vi "SyntaxClean.vi"(8 "error in (no error)":errorcluster, 11 "Logical Parsed Expression":T1) -> (0 "error out":errorcluster, 3 "Logical Parsed Expression Out":T1)   [LabVIEW 2014]
uses:
  TypeDefs/LogicParsedExpression.ctl
  <vilib>/Utility/error.llb/whitespace.ctl
  SeqLoop.lvlib
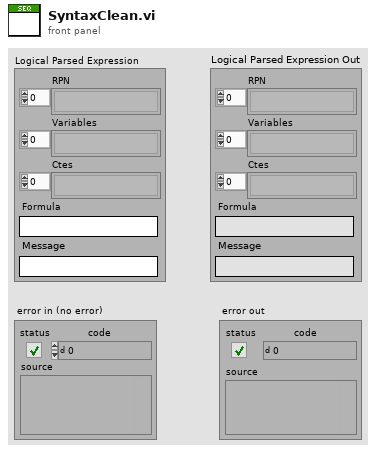
[diagram p1: front panel]
types:
  T1 = typedef "SeqLoop.lvlib/LogicParsedExpression.ctl" = cluster{"RPN ":string[], "Variables":string[], "Ctes":string[], "Formula":string, "Message":string}
  T2 = typedef "whitespace.ctl" = u16
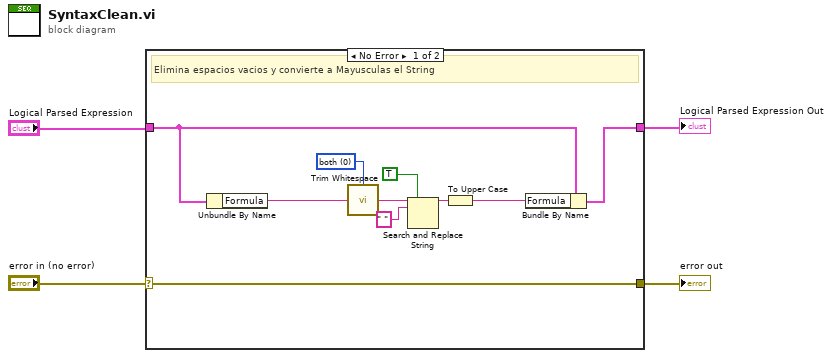
[diagram p0: block diagram]
diagram:
  n1 = case shown="No Error" "error in (no error)" {
    selector: "error in (no error)" -> [w14 w16]
    tunnel: [w14 w16] -> w3
    tunnel: "Logical Parsed Expression" -> [w6 w15]
    tunnel: [w7 w15] -> w2
    frame No Error {
      w13 = T2 0 items=["both", "start of string", "end of string"] ("location (both)")
      # "Elimina espacios vacios y convierte a Mayusculas el String"
      n2 = Unbundle By Name(w6) -> ("Formula"=w8:string)
      n3 = call <vilib>:"Trim Whitespace.vi"("string"=w8, "location (both)"=w13) -> ("trimmed string"=w12:string)
      n4 = Search and Replace String(replace all?=TRUE ("replace all? (F)"), input string=w12, search string=" ") -> (result string=w9:string)  [unwired: 5 in, 3 out]
      n5 = To Upper Case(1:w9) -> (0:w5:string)
      n6 = Bundle By Name(cluster=w6, "Formula"=w5) -> (w7:T1)
    }
    frame Error {
    }
  }
  "error out" <- w3
  "Logical Parsed Expression Out" <- w2
